vi "getStroke.vi"(0 "reference":refnum<class "LineStyle.lvclass">, 5 "error in (no error)":errorcluster) -> (14 "reference out":refnum<class "LineStyle.lvclass">, 15 "lineStyle":T1, 19 "error out":errorcluster)   [LabVIEW 2012, in "LineStyle.lvclass"]
doc: "public Stroke getStroke()"
uses:
  <resource>/Framework/Providers/Open_GDS/UML/LineStyle_class/LineStyle.lvclass
  <resource>/Framework/Providers/Open_GDS/UML/LineStyle_class/LineStyleType.ctl
  <resource>/Framework/Providers/Open_GDS/UML/LineStyle_class/LineStyle.lvclass/LineStyle.ctl
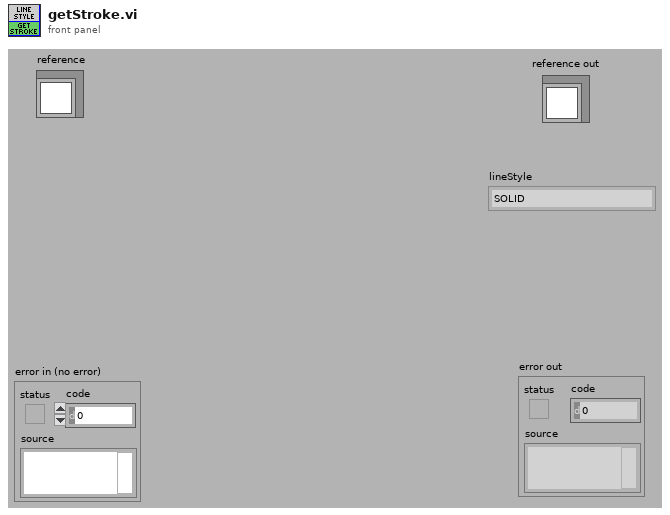
[diagram p1: front panel]
types:
  T1 = typedef "LineStyle.lvclass/LineStyleType.ctl" = enum16{"SOLID", "DOTTED"}
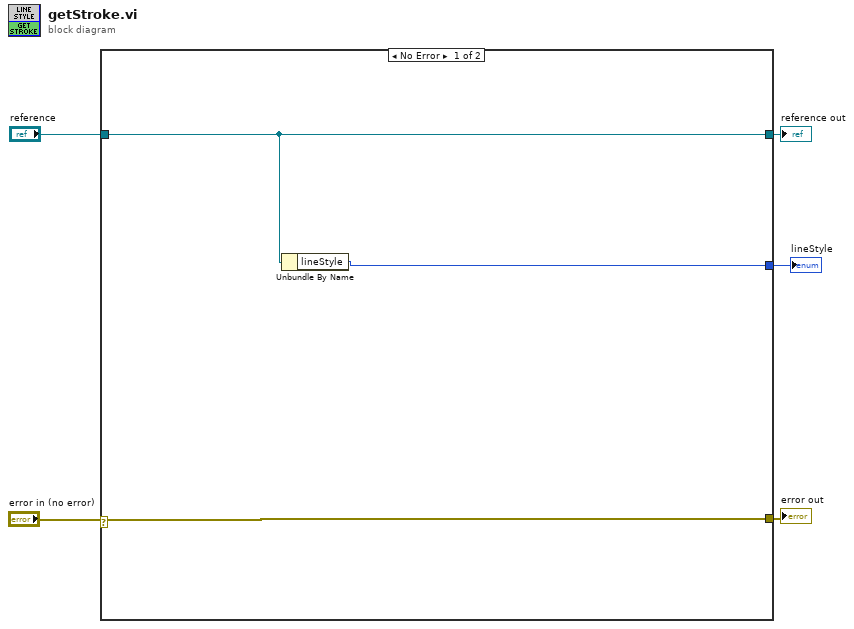
[diagram p0: block diagram]
diagram:
  n1 = case shown="No Error" "error in (no error)" {
    selector: "error in (no error)" -> [w8 w9]
    tunnel: "reference" -> [w7 w10]
    tunnel: [w8 w9] -> w4
    tunnel: [w7 w10] -> w3
    tunnel: [w6 _] -> w1
    frame No Error {
      n2 = Unbundle By Name(w7) -> ("lineStyle"=w6:T1)
    }
    frame Error {
    }
  }
  "reference out" <- w3
  "error out" <- w4
  "lineStyle" <- w1
